vi "Populate_Tree.vi"(0 "Reference_In":refnum<vi>, 5 "File_Path":path, 7 "Parent_Tag":string, 11 "Error_In":errorcluster) -> (4 "Reference_Out":refnum<vi>, 15 "Error_Out":errorcluster={"status"=FALSE, "code"=1088, "source"="Invoke Node in Untitled 1.vi:5370001->Untitled 1.vi:5370002->Untitled 1.vi:5370003->Untitled 1.vi\n<APPEND>\nMethod Name: <b>Edit Tree Items:Add Item</b>"})   [LabVIEW 2023]
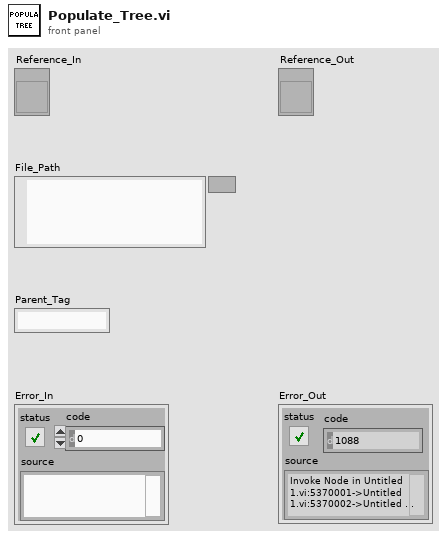
[diagram p1: front panel]
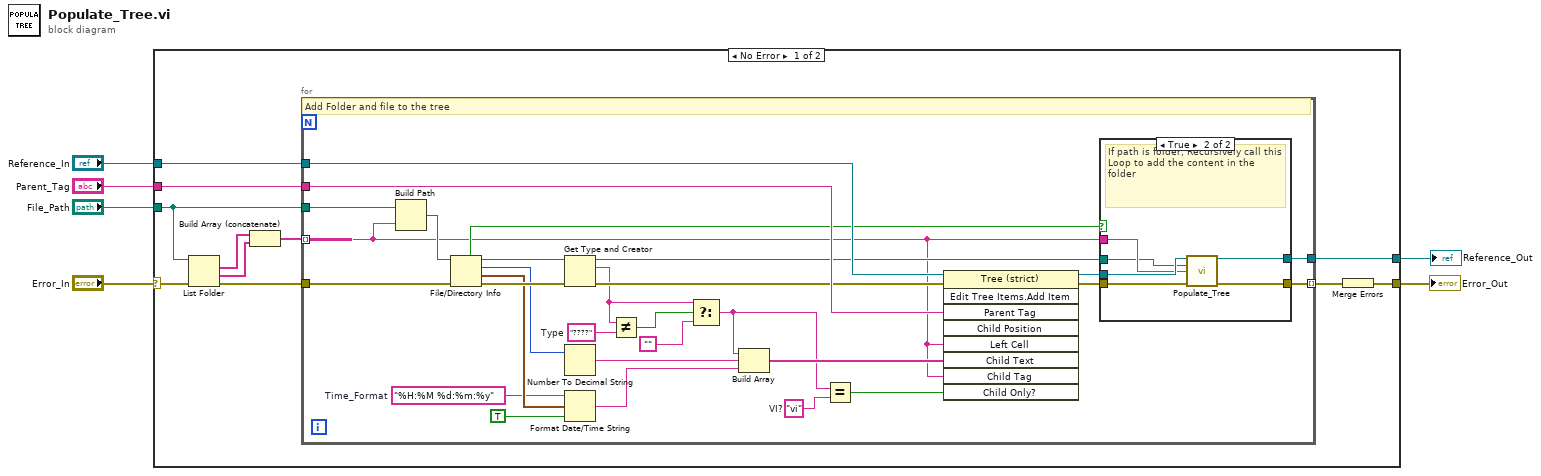
[diagram p0: block diagram]
diagram:
  n1 = case shown="No Error" "Error_In" {
    selector: "Error_In" -> [w8 w56]
    tunnel: "Parent_Tag" -> [w17 _]
    tunnel: "Reference_In" -> [w15 w55]
    tunnel: "File_Path" -> [w10 _]
    tunnel: [w9 w56] -> w3
    tunnel: [w7 w55] -> w1
    frame No Error {
      n2 = List Folder(path=w10, error in=w8) -> (filenames=w12:string[], folder names=w13:string[], error out=w14:errorcluster)  [unwired: 2 in, 1 out]
      n3 = Build Array (concatenate)(w12, w13) -> (w11:string[])
      n4 = for {
        tunnel: w17 -> [w46]
        tunnel: [w45] -> w16 mode=indexing
        tunnel: w14 -> [w44]
        tunnel: w15 -> [w43]
        tunnel: w11 -> [w18] mode=indexing
        tunnel: w10 -> [w25]
        tunnel: [w21] -> w7
        w28 = "????"  # Type
        w31 = "vi"  # VI?
        w32 = "%H:%M %d:%m:%y"  # Time_Format
        # "Add Folder and file to the tree"
        n5 = Build Path(base path=w25, name or relative path=w18) -> (appended path=w20:path)
        n6 = File/Directory Info(path=w20, error in=w44) -> (path out=w41:path, directory=w22:bool, size=w37:i64, last mod=w36:timestamp, error out=w42:errorcluster)  [unwired: 2 out]
        n7 = Get Type and Creator(4:w42, 7:w41) -> (0:w40:errorcluster, 2:w29:string, 3:w19:path)  [unwired: 1 out]
        n8 = Number To Decimal String(number=w37) -> (decimal integer string=w35:string)  [unwired: 1 in]
        n9 = Format Date/Time String(time format string (%c)=w32, seconds (now)=w36, UTC format=TRUE) -> (date/time string=w34:string)
        n10 = Not Equal?(x=w29, y=w28) -> (x != y?=w27:bool)
        n11 = Select(t=w29, s=w27, f="") -> (s? t:f=w26:string)
        n12 = Build Array(w26, w35, w34) -> (w39:string[])
        n13 = Equal?(x=w26, y=w31) -> (x = y?=w38:bool)
        n14 = invoke on="Invoke Node" class="Tree (strict)" method="Edit Tree Items.Add Item"(reference=w43, error in=w40, "Parent Tag"=w46, "Left Cell"=w18, "Child Text"=w39, "Child Tag"=w18, "Child Only?"=w38) -> (reference out=w23:refnum<vi>, error out=w24:errorcluster)  [unwired: 2 in, 7 out]
        n15 = case shown="True" w22 {
          tunnel: [w48 w54] -> w45
          tunnel: w24 -> [w48 w53]
          tunnel: w23 -> [w47 w52]
          tunnel: w19 -> [_ w50]
          tunnel: w18 -> [_ w51]
          tunnel: [w47 w49] -> w21
          frame False {
          }
          frame True {
            # "If path is folder, Recursively call this Loop to add the content in the folder"
            n16 = call "Populate_Tree.vi"("Reference_In"=w52, "File_Path"=w50, "Parent_Tag"=w51, "Error_In"=w53) -> ("Reference_Out"=w49:refnum<vi>, "Error_Out"=w54:errorcluster)  [unwired: 10 in]
          }
        }
      }
      n17 = Merge Errors(w16) -> (w9:errorcluster)
    }
    frame Error {
    }
  }
  "Error_Out" <- w3
  "Reference_Out" <- w1
